vi "3_VNA_KEYSIGHT_rabi_measurements_(Subprog_Rabi).vi"(0 "VNA Power dBm":dbl=-5.0 caption="VNA Power (dBm)" format="%#.3f", 1 "Center Freq (Hz)":dbl=8.586 caption="Center Freq (Hz):" format="%#.6p", 3 "Bandwidth:":dbl=10.0 caption="Bandwidth (1 to 1e6 Hz)" format="%#.3f", 5 "Points:":i32=4 caption="Points", 6 "File name":string="C:\\ExperimentBlue\\Photon_Source_Dec8'17\\Photon_Source_Dec8'17_Q_osc_05CAL", 7 "Comments":string=" cell Ay\nI=0.0082mA \nf=6.93602GHz\nPulse length sweep 1.5 to 51.5 ns 251 points\nPower  10 to -15 dBm 5 points \nKeysight frequency of pulse generator 10MHz ( 100ns pulse to pulse) \nbandwidth 5Hz\nTransmission Input (VNA):  -chopper1-20-40(4K)\nOut: ~+35dB(4K)+35(RT)", 8 "Start (ns)":dbl=2.0, 9 "End (ns)":dbl=52.0, 10 "Numeric":u32=251, 11 "save":bool, 12 "Gen Power (dBm)":dbl format="%#.3f", 13 "Gen Freq (Hz)":dbl=10905300000.0 caption="Gen Freq:" format="%^#.6e") -> ()   [LabVIEW 2013]
uses:
  <vilib>/Analysis/baseanly.llb/Mean (DBL).vi
  <vilib>/Analysis/NI_AALBase.lvlib
panel:
  out "Index Selection":dbl[](graph)
  in  "Index selection":i32
  in  "Outputs":T1={"Ouput 1"=TRUE, "Ouput 2"=FALSE, "Ouput 1 Neg"=FALSE, "Ouput 2 Neg"=FALSE}
  in  "Frequency Parameters":T2={"Coupling"=FALSE, "Frequency 2 (MHz)"=2.0, "Frequency 1 (MHz)"=10.0, "WAVEFORM"=enum."PULSE"} {"Frequency 1 (MHz)" min=0.0 max=14.5; "Frequency 2 (MHz)" min=0.0 max=14.5}
  in  "Connection":T3={"Type"=1, "VISA"="TCPIP0::192.168.0.8::inst0::INSTR", "GPIB"="10"} {"Type" items=["VISA", "GPIB"]}
  out "(Current)":i32
  in  "?":enum32{"VNA", "Generator"}(tab)
  in  "?":enum32{"Page 1", "Page 2"}(tab)
  out "Pow":dbl=34.32006687269598
  in  "Tab Control":enum32{"Page 1", "Page 2"}(tab)
  in  "Save?":bool
  in  "Name":string="data_labView_Photon_Source_Mar9'18_temp"
  out "Waveform Graph":dbl[][](graph)=[[0.019127955194562674, 0.0207779030315578, 0.02240485232323408, 0.024474252481013536, 0.02520590042695403, 0.02643036050722003, 0.027151720132678747, 0.028597308322787285, 0.029717680998146534, 0.03038754453882575, 0.030780285131186247, 0.031893023289740086, 0.0323828961700201, 0.03328412305563688, 0.034057945013046265, 0.034034344367682934, 0.034477829933166504, 0.03534907568246126, 0.03493230417370796, 0.03513764310628176, 0.03533593285828829, 0.03527460992336273, 0.03569782059639692, 0.035154384560883045, 0.035424877889454365, 0.03494449704885483, 0.03477480635046959, 0.03458270337432623, 0.03402741812169552, 0.03313762880861759, 0.03322163317352533, 0.032859284430742264, 0.032248022966086864, 0.031421750318259, 0.030632789712399244, 0.0297507313080132, 0.029253825079649687, 0.028674961533397436, 0.027543761767446995, 0.027653961442410946, 0.02601017616689205, 0.02603383781388402, 0.024602124467492104, 0.023599382489919662, 0.022910801228135824, 0.02219532523304224, 0.020895992871373892, 0.02001399314031005, 0.019471243023872375, 0.01872662967070937, 0.017840758431702852, 0.017276559490710497, 0.01574999885633588, 0.015208411030471325, 0.014366974821314216, 0.013177897548303008, 0.012374990619719028, 0.011526171816512942, 0.010659741004928946, 0.01052671717479825, 0.00935881887562573, 0.008008884848095477, 0.0082545563345775, 0.007215638877823949, 0.006160384742543101, 0.006210934603586793, 0.004838436841964722, 0.0045333654852584004, 0.004386340617202222, 0.0034725037985481326, 0.0031686159782111645, 0.002354342199396342, 0.0015043105813674629, 0.0009552944247843697, 0.0007856405572965743, 0.0002383617647865319, -1.9010731193702817e-05, 0.0002983270533150063, -0.0009187151190417355, -0.0012520845011749768, -0.00017930776266439358, -0.0015206103125819936, -0.001488478374085389, -0.0010812451073434204, -0.0014266804791986947, -0.0014832954620942473, -0.0014105267982813532, -0.0009959812159650028, -0.00080056679144036, -0.0012878108827862889, -0.0006374359654728324, -0.00026426462090967123, -0.0001149393829109612, -1.0142728569917476e-05, 0.0006734268172294833, 0.0012570339313242584, 0.0016542751400265843, 0.0027212004060857, 0.001964373601367697, 0.0030421327683143318, 0.003769123402889818, 0.004313481156714261, 0.004636538971681148], [-0.01108602387830615, -0.011888890760019422, -0.013314370764419436, -0.013788532000035048, -0.014694856014102697, -0.01534495665691793, -0.015825830632820725, -0.016432047821581364, -0.016871558502316475, -0.017548938747495413, -0.01813248498365283, -0.01837828289717436, -0.018622552044689652, -0.019042819272726774, -0.01926602888852358, -0.019426763989031315, -0.01968517294153571, -0.020793242380023003, -0.020589482970535755, -0.020488033071160316, -0.020475211087614298, -0.020613223779946566, -0.02047412795946002, -0.020636729430407286, -0.020122316665947437, -0.020187079906463623, -0.019573011435568333, -0.019980215933173895, -0.019262139685451984, -0.018981218338012695, -0.018678490072488785, -0.018447216600179672, -0.018502402119338512, -0.0174516923725605, -0.01674525486305356, -0.017023920081555843, -0.0162105830386281, -0.015761795919388533, -0.01474237465299666, -0.014489330118522048, -0.013798840343952179, -0.013845508452504873, -0.013231844874098897, -0.01217434392310679, -0.011762261390686035, -0.010876467218622565, -0.010729442117735744, -0.009808138478547335, -0.0095574373845011, -0.008999691344797611, -0.00815515429712832, -0.007421280490234494, -0.007225316716358066, -0.006310812779702246, -0.006102788727730513, -0.004980261554010212, -0.00442964251851663, -0.004131958994548768, -0.003192006377503276, -0.003015937574673444, -0.0023254714033100754, -0.0024703676463104784, -0.0015535818674834445, -0.0012101363390684128, -3.334921711939388e-05, 4.7374960558954653e-05, 0.0003741370237548835, 0.0008621039160061627, 0.0013745578180532902, 0.0012972068507224321, 0.0021619122417178005, 0.003051207691896707, 0.002743339806329459, 0.0028674471541307867, 0.0036189278471283615, 0.003626895137131214, 0.0041286274790763855, 0.00398181367199868, 0.004171250620856881, 0.004108947701752186, 0.004871417535468936, 0.004986890591681004, 0.004586611641570926, 0.005213201860897243, 0.004767011036165059, 0.005303648067638278, 0.005151833640411496, 0.004916338250041008, 0.005461058346554637, 0.005141314351931214, 0.004757799790240824, 0.004543771967291832, 0.004539029439911246, 0.0042993074748665094, 0.003856932569760829, 0.0034965855884365737, 0.003723626199644059, 0.003367167024407536, 0.0033197872107848525, 0.0027364877169020474, 0.002761686861049384, 0.0017728788079693916, 0.0019938760669901967], [0.02210833768865428, 0.023938817387091076, 0.02606242269011756, 0.028091148948029658, 0.0291766380792704, 0.030561931407296662, 0.03142726239082939, 0.03298208966877775, 0.03417294324761458, 0.03509085513723575, 0.03572412300448424, 0.03680932241713334, 0.03735574131262124, 0.03834660106758502, 0.039129573057281215, 0.03918846457343736, 0.039701722766632204, 0.0410111701890931, 0.04054864589451091, 0.040674481707692216, 0.040839471348779986, 0.040855882071588606, 0.04115245206585973, 0.04076402035420808, 0.04074100638775899, 0.04035636342818033, 0.03990476078577027, 0.03993960942989917, 0.039101089617689135, 0.038188860845186676, 0.03811250322537659, 0.03768331691338178, 0.03717894389848867, 0.035942842955580125, 0.0349109061181845, 0.03427710414117268, 0.033445018825573984, 0.03272136350377648, 0.031240941450461975, 0.03121990183747959, 0.02944379831255882, 0.029486587046113042, 0.027934678216979533, 0.026554575949610155, 0.025753749356898954, 0.024716998227096526, 0.023489645511125753, 0.02228810224839115, 0.021690410652022193, 0.02077693680804554, 0.019616299422376967, 0.018803055920535737, 0.01732823319401793, 0.01646578646807419, 0.015609420097223064, 0.014087582792655476, 0.013143900702606678, 0.012244415946724846, 0.011127397854223833, 0.010950235336855532, 0.009643407488765647, 0.008381226212076064, 0.008399483132889005, 0.007316411304341655, 0.006160475009805681, 0.006211115281245374, 0.004852880545225249, 0.004614610036062125, 0.004596671970598881, 0.003706889294879525, 0.003835882135606408, 0.003853932481368613, 0.0031287159695641705, 0.0030223898854642903, 0.0037032242502973525, 0.003634719338086257, 0.004128671247373076, 0.003992973722585114, 0.004271225727113329, 0.004295482139855451, 0.004874716410072072, 0.005213572047658613, 0.004822092307361383, 0.005324149192558052, 0.004975923171497534, 0.005507163358139345, 0.005341439478936873, 0.00501620976150035, 0.005519426188656858, 0.005300148123892075, 0.004800310766408141, 0.004551450261247684, 0.004540484480551052, 0.00429931943897937, 0.003915281921630383, 0.0037156755888751725, 0.004074557437757582, 0.004329289251174894, 0.003857427999411132, 0.004091813388316676, 0.004672601582063735, 0.004663605789201738, 0.005047081870391481]]
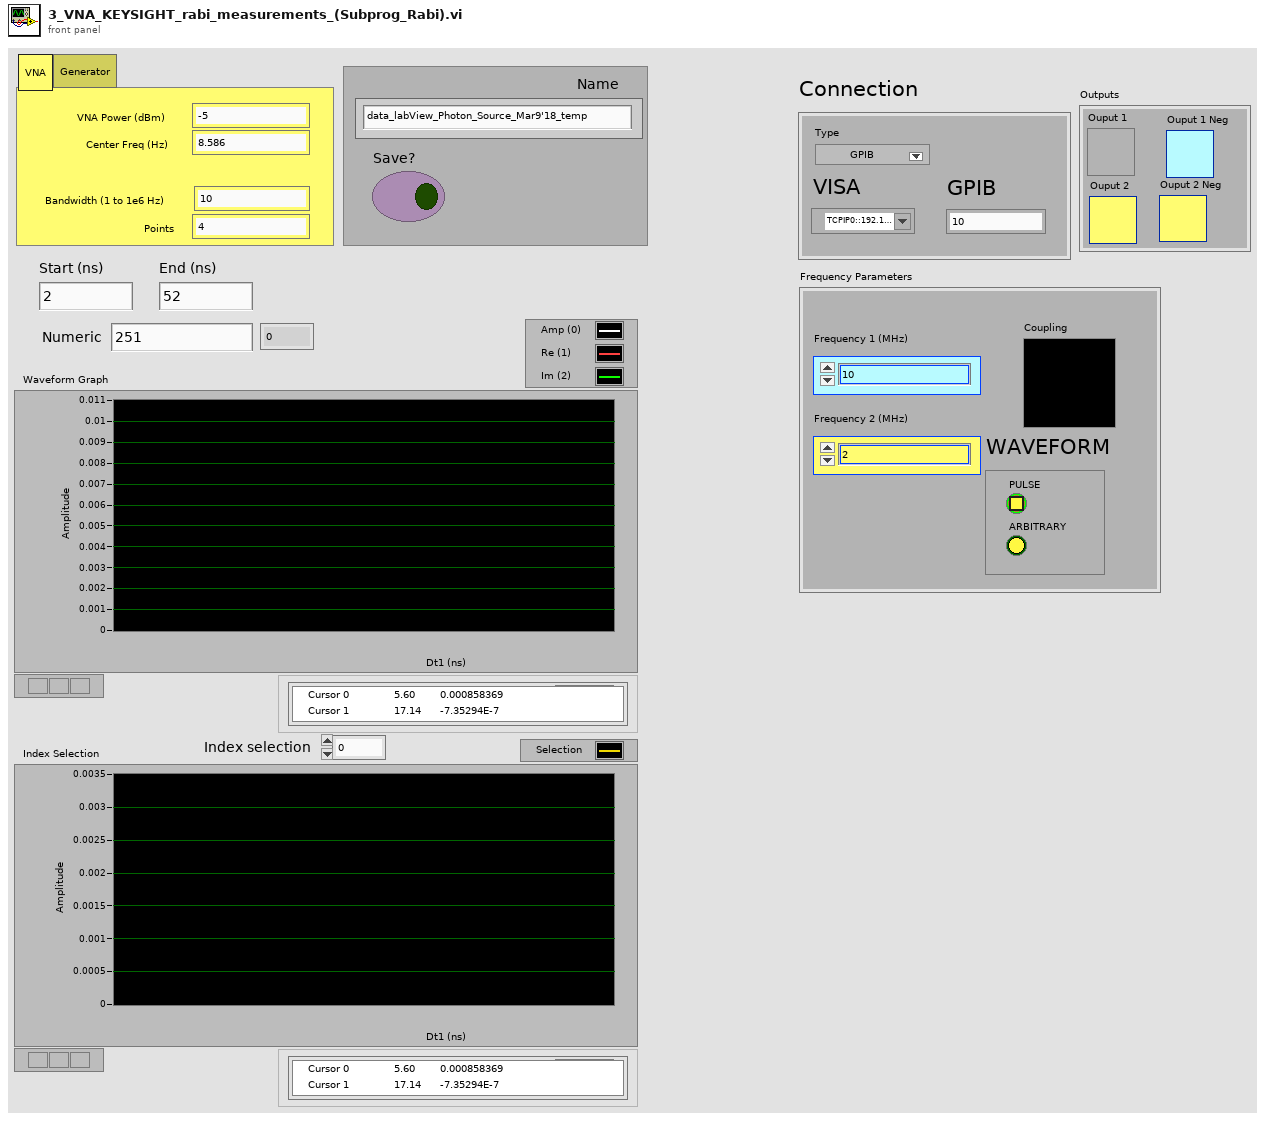
[diagram p1: front panel]
types:
  T1 = cluster{"Ouput 1":bool, "Ouput 2":bool, "Ouput 1 Neg":bool, "Ouput 2 Neg":bool}
  T2 = cluster{"Coupling":bool, "Frequency 2 (MHz)":dbl, "Frequency 1 (MHz)":dbl, "WAVEFORM":enum32{"PULSE", "ARBITRARY"}}
  T3 = cluster{"Type":u16, "VISA":refnum<visa-resource-name>, "GPIB":string}
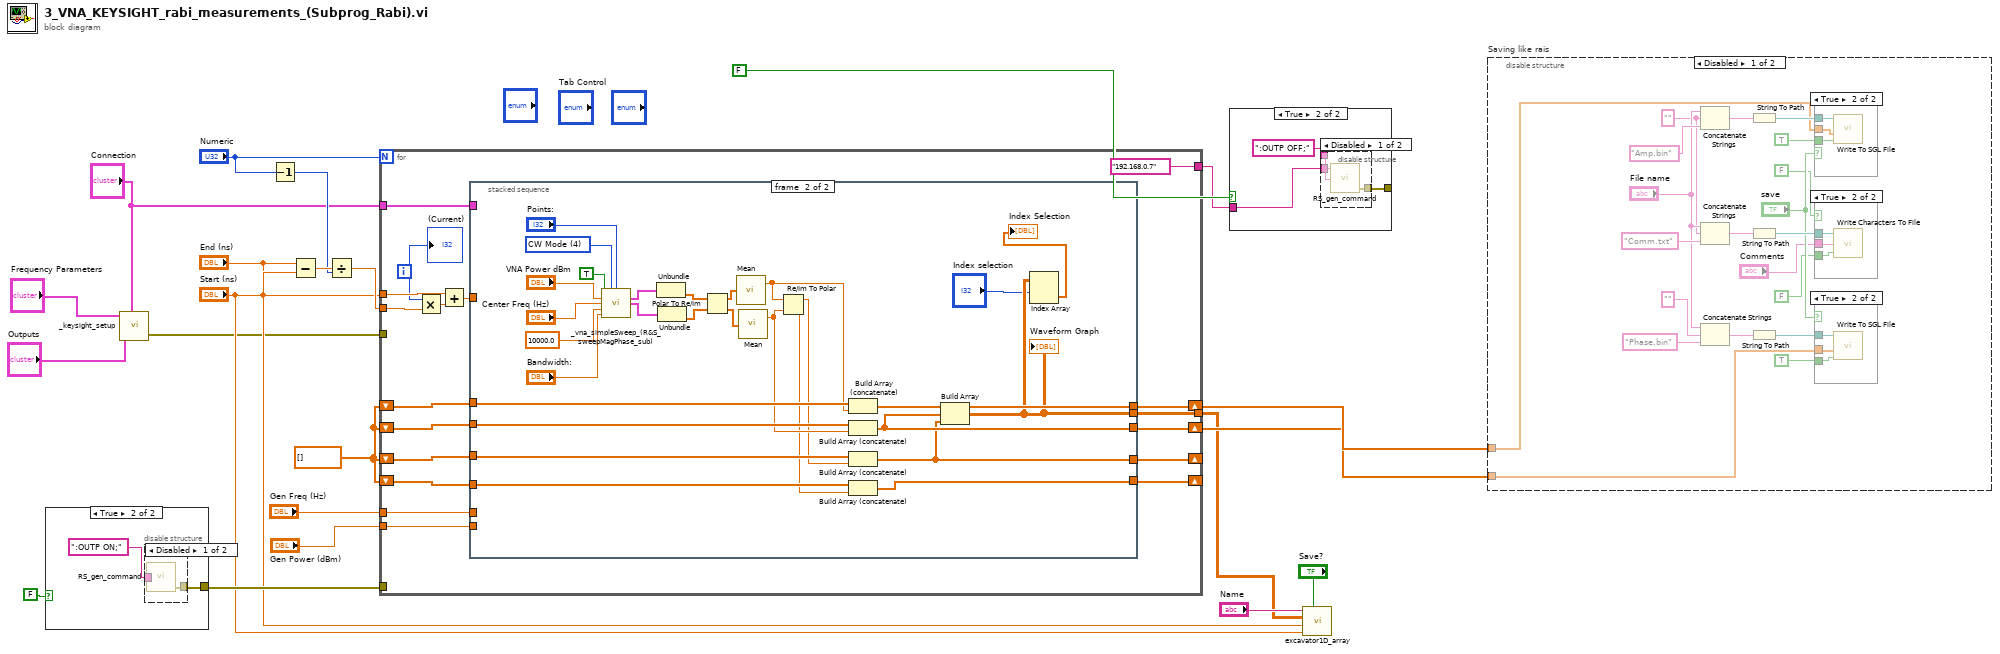
[diagram p0: block diagram]
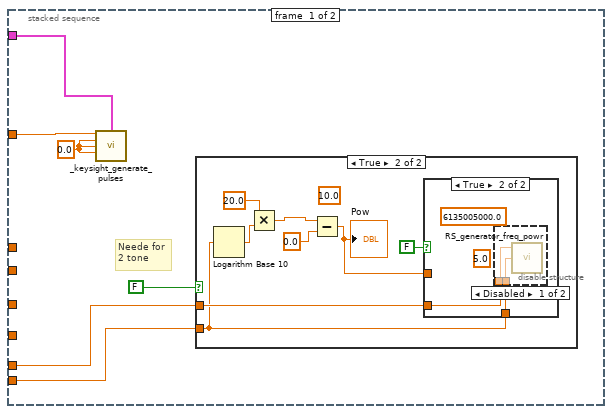
[diagram p10: hidden frame]
diagram:
  w10 = dbl[] []
  n1 = case shown="True" FALSE {
    tunnel: [_ w23] -> w15
    frame False {
    }
    frame True {
      n2 = disable-structure shown="Disabled" {
        disable-tunnel: ":OUTP ON;" -> [w26 _]
        disable-tunnel: [w25 _] -> w23
        frame Disabled {
          n3 = call "RS_gen_command.vi"("Comand"=w26) -> ("error out"=w25:errorcluster)  [unwired: 4 in]
        }
        frame Enabled {
        }
      }
    }
  }
  n4 = call "_keysight_setup.vi"("Frequency Parameters"="Frequency Parameters", "Outputs"="Outputs", "Keysight Connection"="Connection") -> ("error out"=w1:errorcluster)  [unwired: 3 in]
  n5 = Decrement(x="Numeric") -> (x-1=w20:u32)
  n6 = Subtract(x="End (ns)", y="Start (ns)") -> (x-y=w21:dbl)
  n7 = Divide(x=w21, y=w20) -> (x/y=w19:dbl)
  n8 = for {
    N: "Numeric" -> [_]
    tunnel: w19 -> [w29]
    tunnel: "Start (ns)" -> [w43]
    shift-right: [w41] -> w12
    shift-left: w10 -> [w42]
    shift-right: [w39] -> w11
    shift-left: w10 -> [w40]
    shift-right: [w38] -> _
    shift-left: w10 -> [w37]
    tunnel: "Gen Power (dBm)" -> [w35]
    tunnel: "Gen Freq (Hz)" -> [w34]
    tunnel: w15 -> [_]
    tunnel: ["192.168.0.7" ("address")] -> w13
    shift-right: [w31] -> _
    shift-left: w10 -> [w32]
    tunnel: [w30] -> w7
    tunnel: "Connection" -> [w27]
    tunnel: w1 -> [_]
    i -> [w28]
    n9 = Multiply(x=w28, y=w29) -> (x*y=w44:dbl)
    n10 = Add(x=w43, y=w44) -> (x+y=w36:dbl)
    n11 = stacked-sequence {
      tunnel: w42 -> [_ w90]
      tunnel: [_ w82] -> w41
      tunnel: w40 -> [_ w85]
      tunnel: [_ w81] -> w39
      tunnel: [_ w79] -> w38
      tunnel: w37 -> [_ w80]
      tunnel: w36 -> [w47 _]
      tunnel: w35 -> [w50 _]
      tunnel: w34 -> [w49 _]
      tunnel: w32 -> [_ w77]
      tunnel: [_ w75] -> w31
      tunnel: [_ w65] -> w30
      tunnel: w27 -> [w45 _]
      frame #0 {
        w46 = 0.0 ("Ch2 pulse_delay (ns)")
        # "Neede for\n2 tone"
        n12 = call "_keysight_generate_pulses.vi"("Ch1 pulse_width (ns)"=w47, "Connection"=w45, "Ch2 pulse_width (ns)"=w46, "Ch1 pulse_delay (ns)"=w46, "Ch2 pulse_delay (ns)"=w46) -> ()  [unwired: 9 in, 2 out]
        n13 = case shown="True" FALSE {
          tunnel: w50 -> [_ w51]
          tunnel: w49 -> [_ w52]
          frame False {
          }
          frame True {
            (unwired) 10.0
            n14 = Logarithm Base 10(1:w51) -> (0:w57:dbl)
            n15 = Multiply(x=20.0, y=w57) -> (x*y=w55:dbl)
            n16 = Subtract(x=w55, y=0.0) -> (x-y=w53:dbl)
            "Pow" <- w53
            n17 = case shown="True" FALSE {
              tunnel: w53 -> [_ _]
              tunnel: w51 -> [_ w60]
              tunnel: w52 -> [_ w59]
              frame False {
              }
              frame True {
                (unwired) 5.0 ("Power  (dBm)")
                (unwired) 6135005000.0 ("F (GHz)")
                n18 = disable-structure shown="Disabled" {
                  disable-tunnel: w60 -> [w61 _]
                  disable-tunnel: w59 -> [w62 _]
                  frame Disabled {
                    n19 = call "RS_generator_freq_powr.vi"("Power (dBm)"=w61, "Frequnecy (Hz)"=w62) -> ()  [unwired: 1 in, 2 out]
                  }
                  frame Enabled {
                  }
                }
              }
            }
          }
        }
      }
      frame #1 {
        w68 = 4 items=["Lin. Frequency", "Log. Frequency", "Segmented Frequency", "Power", "CW Mode", "Time"] ("Sweep Type")
        n20 = call "_vna_simpleSweep_(R&S_sweepMagPhase_sub).vi"("Boolean"=TRUE, "Sweep Type"=w68, "Points:"="Points:", "Power dBm"="VNA Power dBm", "Center Freq:"="Center Freq (Hz)", "Span Freq:"=10000.0, "Bandwidth:"="Bandwidth:") -> ("Lin Mag"=w66:cluster{dbl[], dbl[]}, "Phase"=w67:cluster{dbl[], dbl[]})  [unwired: 7 in]
        n21 = Unbundle(w66) -> (w89:dbl[])  [unwired: 1 out]
        n22 = Unbundle(w67) -> (w88:dbl[])  [unwired: 1 out]
        n23 = Polar To Re/Im(2:w88, 3:w89) -> (0:w86:dbl[], 1:w87:dbl[])
        n24 = call-poly <vilib>:"Mean.vi"("X"=w87) -> ("mean"=w83:dbl)  [unwired: 1 out]
        n25 = call-poly <vilib>:"Mean.vi"("X"=w86) -> ("mean"=w84:dbl)  [unwired: 1 out]
        n26 = Re/Im To Polar(2:w84, 3:w83) -> (0:w76:dbl, 1:w78:dbl)
        n27 = Build Array (concatenate)(w90, w83) -> (w82:dbl[])
        n28 = Build Array (concatenate)(w85, w84) -> (w81:dbl[])
        n29 = Build Array (concatenate)(w80, w78) -> (w79:dbl[])
        n30 = Build Array (concatenate)(w77, w76) -> (w75:dbl[])
        n31 = Build Array(w82, w81, w79) -> (w65:dbl[][])
        "Waveform Graph" <- w65
        n32 = Index Array(array=w65, index (row)="Index selection") -> (element=→"Index Selection":dbl[])  [unwired: 1 in]
      }
    }
    "(Current)" <- w28
  }
  n33 = case shown="True" FALSE {
    tunnel: [_ w92] -> _
    tunnel: w13 -> [_ w91]
    frame False {
    }
    frame True {
      n34 = disable-structure shown="Disabled" {
        disable-tunnel: ":OUTP OFF;" -> [w96 _]
        disable-tunnel: [w95 _] -> w92
        disable-tunnel: w91 -> [w94 _]
        frame Disabled {
          n35 = call "RS_gen_command.vi"("Comand"=w96, "address"=w94) -> ("error out"=w95:errorcluster)  [unwired: 3 in]
        }
        frame Enabled {
        }
      }
    }
  }
  n36 = call "excavator1D_array.vi"("Name"="Name", "Array"=w7, "x_max"="End (ns)", "x_min"="Start (ns)", "Save?"="Save?") -> ()  [unwired: 1 out]
  n37 = disable-structure "Saving like rais" shown="Disabled" {
    disable-tunnel: w12 -> [w98 _]
    disable-tunnel: w11 -> [w97 _]
    frame Disabled {
      w100 = "" ("format string")
      n38 = Concatenate Strings("File name", w100, "Amp.bin") -> (w114:string)
      n39 = Concatenate Strings("File name", w100, "Comm.txt") -> (w107:string)
      n40 = Concatenate Strings("File name", "" ("format string"), "Phase.bin") -> (w110:string)
      n41 = String To Path(string=w114) -> (path=w116:path)
      n42 = String To Path(string=w107) -> (path=w104:path)
      n43 = String To Path(string=w110) -> (path=w112:path)
      n44 = case shown="True" "save" {
        tunnel: w116 -> [_ w125]
        tunnel: w98 -> [_ w124]
        tunnel: TRUE -> [_ w123]
        frame False {
        }
        frame True {
          n45 = call <vilib>:"Write To SGL File.vi"("append to file? (new file:F)"=w123, "1D array"=w124, "file path (dialog if empty)"=w125) -> ()  [unwired: 4 in, 1 out]
        }
      }
      n46 = case shown="True" FALSE {
        tunnel: w104 -> [_ w119]
        tunnel: "Comments" -> [_ w118]
        tunnel: FALSE -> [_ w117]
        frame False {
        }
        frame True {
          n47 = call <vilib>:"Write Characters To File.vi"("append to file? (new file:F)"=w117, "character string"=w118, "file path (dialog if empty)"=w119) -> ()  [unwired: 2 in, 1 out]
        }
      }
      n48 = case shown="True" "save" {
        tunnel: w112 -> [_ w122]
        tunnel: w97 -> [_ w121]
        tunnel: TRUE -> [_ w120]
        frame False {
        }
        frame True {
          n49 = call <vilib>:"Write To SGL File.vi"("append to file? (new file:F)"=w120, "1D array"=w121, "file path (dialog if empty)"=w122) -> ()  [unwired: 4 in, 1 out]
        }
      }
    }
    frame Enabled {
    }
  }
